vi "ac1.vi"(0 "V1":dbl, 5 "V1 angle":dbl, 7 "R1":dbl, 9 "C1":dbl, 12 "L1":dbl) -> (2 "Zt":dbl, 3 "Zt angle":dbl, 4 "I":dbl, 6 "I angle":dbl, 8 "Vr":dbl, 10 "Vr angle":dbl, 13 "Vl angle":dbl, 14 "Vl":dbl)   [LabVIEW 2018]
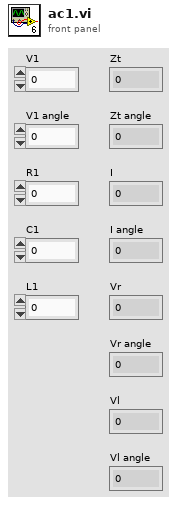
[diagram p1: front panel]
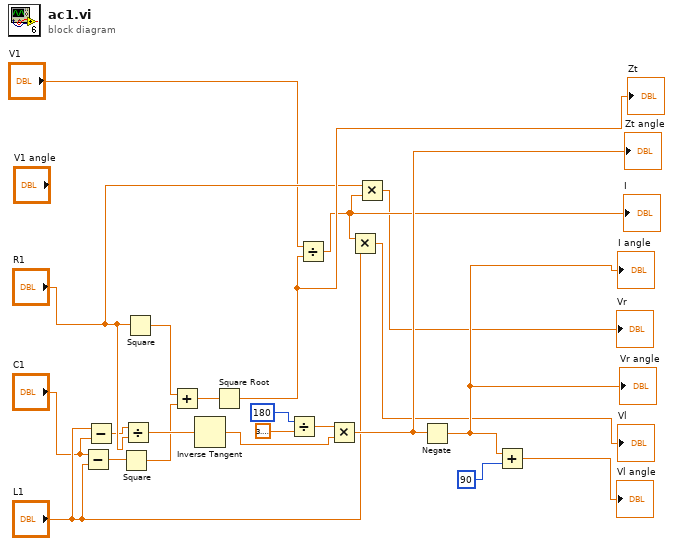
[diagram p0: block diagram]
diagram:
  n1 = Subtract(x="C1", y="L1") -> (x-y=w1:dbl)
  n2 = Subtract(x="L1", y="C1") -> (x-y=w7:dbl)
  n3 = Square(x=w1) -> (x^2=w3:dbl)
  n4 = Divide(x=w7, y="R1") -> (x/y=w8:dbl)
  n5 = Square(x="R1") -> (x^2=w2:dbl)
  n6 = Add(x=w2, y=w3) -> (x+y=w4:dbl)
  n7 = Inverse Tangent(1:w8) -> (0:w12:dbl)
  n8 = Square Root(x=w4) -> (sqrt(x)=w18:dbl)
  "Zt" <- w18
  n9 = Divide(x=180, y=3.141592653589793) -> (x/y=w11:dbl)
  n10 = Divide(x="V1", y=w18) -> (x/y=w15:dbl)
  "I" <- w15
  n11 = Multiply(x=w11, y=w12) -> (x*y=w19:dbl)
  "Zt angle" <- w19
  n12 = Multiply(x=w15, y="L1") -> (x*y=→"Vl":dbl)
  n13 = Multiply(x="R1", y=w15) -> (x*y=→"Vr":dbl)
  n14 = Negate(x=w19) -> (-x=w21:dbl)
  "I angle" <- w21
  "Vr angle" <- w21
  n15 = Add(x=w21, y=90) -> (x+y=→"Vl angle":dbl)
